vi "Global Schedule Selector.vi"(6 "Scheduler In":refnum<class "Scheduler.lvclass">, 7 "Objective":T1, 8 "error in (no error)":errorcluster, 9 "Reorder?":bool, 10 "Schedule in":u16[](array[numeric]), 11 "OSSP_Problem in":refnum<class "OSSP_Problem.lvclass">) -> (0 "error out":errorcluster, 1 "Total Tardiness or Makespan (U16)":u16, 2 "Schedule out":u16[](array[numeric]), 3 "OSSP_Problem out":refnum<class "OSSP_Problem.lvclass">, 4 "Scheduler out":refnum<class "Scheduler.lvclass">)   [LabVIEW 2013]
uses:
  Classes/OSSP_Problem.lvclass
  GA/Controls/Objective.ctl
  Classes/Scheduler.lvclass
  Classes/Scheduler.lvclass/Scheduler.ctl
  Classes/OSSP_Problem.lvclass/OSSP_Problem.ctl
  Classes/Scheduler_Class/Operation to Machine Job Tuple.vi
  Classes/Scheduler_Class/Prins FIFO Scheduler Methods and Controls/Prins FIFO Scheduler.vi
  Classes/Scheduler_Class/Prins FIFO Scheduler Methods and Controls/Methods/Calculate Final Completion Times of Jobs.vi
  Classes/Scheduler_Class/Prins FIFO Scheduler Methods and Controls/Methods/Reorder Schedule(Prins FIFO) based on Start Times.vi
  Classes/Scheduler_Class/Modified GT Active Scheduler/GT Find Subset of Operations.vi
  Classes/Scheduler_Class/Modified GT Active Scheduler/Select Operation to Schedule Based on Rule.vi
  Classes/Scheduler_Class/Prins FIFO Scheduler Methods and Controls/Methods/UpdateMachineGaps.vi
  Classes/Scheduler_Class/Prins FIFO Scheduler Methods and Controls/Methods/UpdateJobGaps.vi
  Classes/Scheduler_Class/Prins FIFO Scheduler Methods and Controls/Methods/Find Intersecting Gaps.vi
  Classes/Scheduler_Class/GT Algorithm Find M_ok and J_ok.vi
  Classes/Scheduler_Class/Prins FIFO Scheduler Methods and Controls/Methods/Transform to Plain Job and Machine Gaps Array.vi
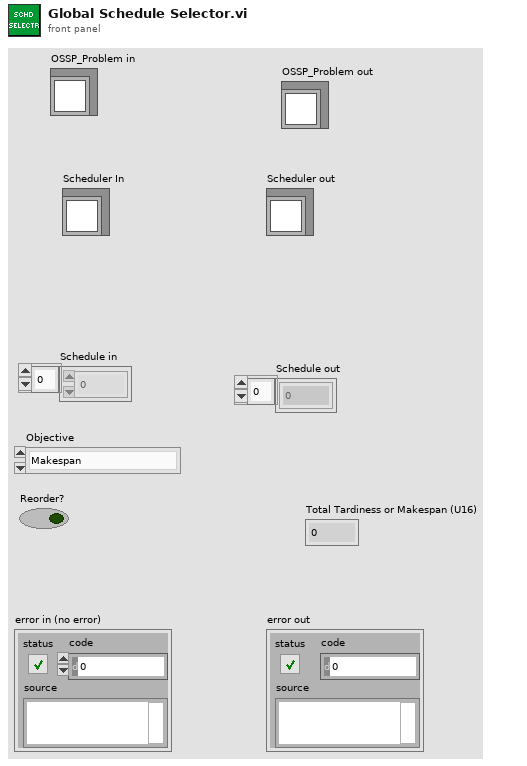
[diagram p1: front panel]
types:
  T1 = typedef "Objective.ctl" = enum16{"Makespan", "Total Tardiness"}
  T2 = typedef "Scheduler Type.ctl" = enum16{"Non Delay Scheduler", "GT Active Scheduler", "My Faulty Scheduler", "Prins FIFO Scheduler", "SemiActive Scheduler", "Modified GT Scheduler"}
  T3 = typedef "Scheduler.lvclass/Operation Selection Rule from Subset to Schedule.ctl" = enum16{"First Operation in Order", "SPT", "EDD", "MDD"}
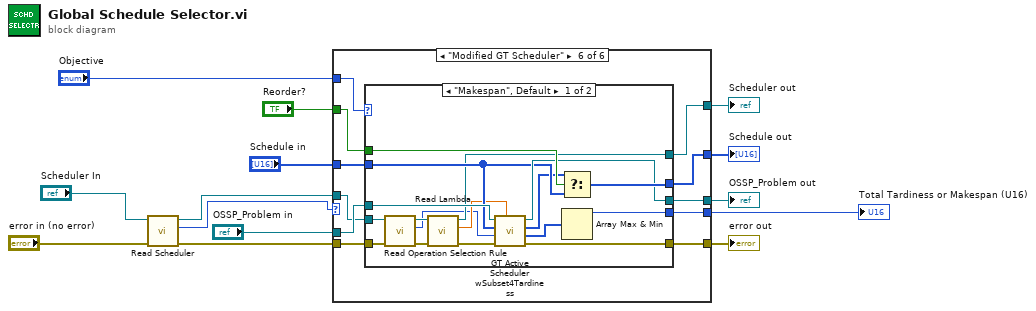
[diagram p0: block diagram]
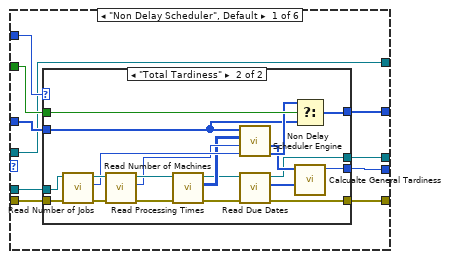
[diagram p2: hidden frame]
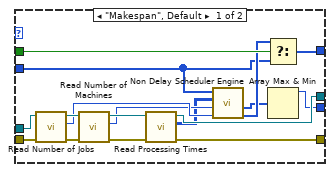
[diagram p3: hidden frame]
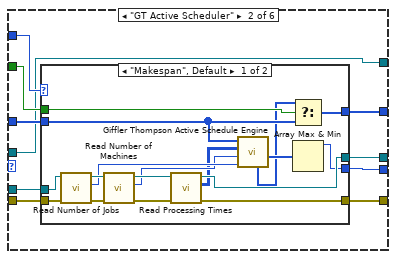
[diagram p4: hidden frame]
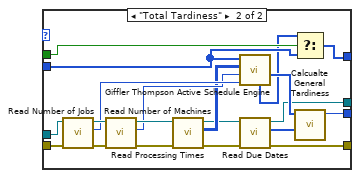
[diagram p5: hidden frame]
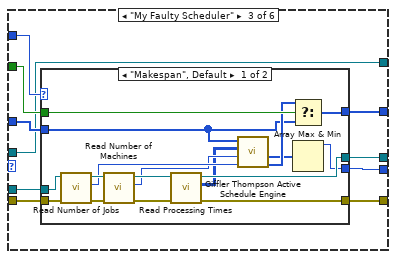
[diagram p6: hidden frame]
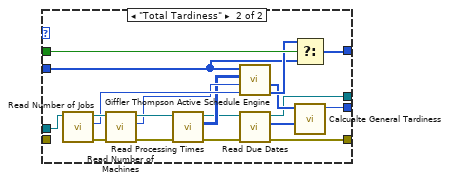
[diagram p7: hidden frame]
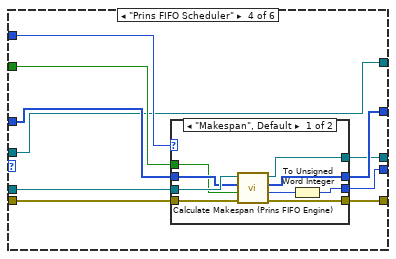
[diagram p8: hidden frame]
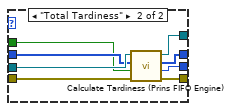
[diagram p9: hidden frame]
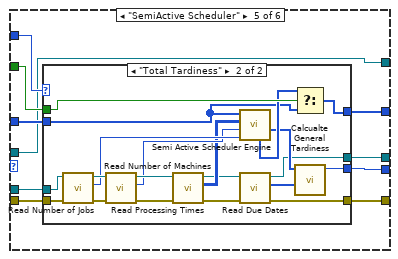
[diagram p10: hidden frame]
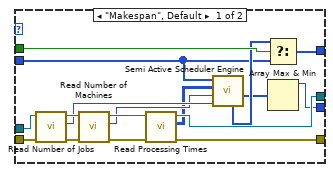
[diagram p11: hidden frame]
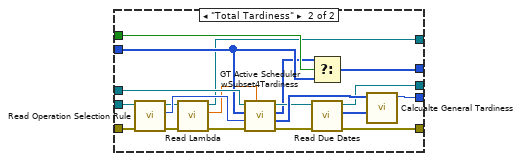
[diagram p12: hidden frame]
diagram:
  n1 = call "Read Scheduler.vi"("error in (no error)"="error in (no error)", "Scheduler in"="Scheduler In") -> ("error out"=w4:errorcluster, "Scheduler"=w1:T2, "Scheduler out"=w2:refnum<class "Scheduler.lvclass">)  [unwired: 7 in]
  n2 = case shown="\"Modified GT Scheduler\"" w1 {
    tunnel: [w16 w66 w111 w164 w184 w232] -> w7
    tunnel: "Schedule in" -> [w19 w69 w117 w163 w190 w238]
    tunnel: [w17 w65 w112 w162 w185 w233] -> w9
    tunnel: "Objective" -> [w24 w63 w115 w161 w189 w237]
    tunnel: "Reorder?" -> [w18 w68 w114 w160 w187 w235]
    tunnel: [w22 w64 w110 w159 w183 w231] -> w12
    tunnel: "OSSP_Problem in" -> [w23 w70 w118 w158 w191 w239]
    tunnel: w4 -> [w21 w71 w116 w157 w188 w236]
    tunnel: [w20 w67 w113 w156 w186 w234] -> w14
    tunnel: w2 -> [w15 w62 w109 w155 w182 w230]
    tunnel: [w15 w62 w109 w155 w182 w229] -> w6
    frame "Non Delay Scheduler", Default {
      n3 = case shown="\"Total Tardiness\"" w24 {
        tunnel: w23 -> [w41 w61]
        tunnel: [w38 w45] -> w22
        tunnel: w21 -> [w37 w58]
        tunnel: [w34 w44] -> w20
        tunnel: w19 -> [w28 w50]
        tunnel: w18 -> [w30 w52]
        tunnel: [w27 w49] -> w17
        tunnel: [w25 w42] -> w16
        frame "Makespan", Default {
          n4 = call "Read Number of Jobs.vi"("error in (no error)"=w37, "OSSP_Problem in"=w41) -> ("error out"=w36:errorcluster, "Number of Jobs"=w33:i32, "OSSP_Problem out"=w40:refnum<class "OSSP_Problem.lvclass">)  [unwired: 7 in]
          n5 = call "Read Number of Machines.vi"("error in (no error)"=w36, "OSSP_Problem in"=w40) -> ("error out"=w35:errorcluster, "Number of Machines"=w32:i32, "OSSP_Problem out"=w39:refnum<class "OSSP_Problem.lvclass">)  [unwired: 7 in]
          n6 = call "Read Processing Times.vi"("error in (no error)"=w35, "OSSP_Problem in"=w39) -> ("error out"=w34:errorcluster, "Processing Times"=w31:u16[][], "OSSP_Problem out"=w38:refnum<class "OSSP_Problem.lvclass">)  [unwired: 7 in]
          n7 = call "Non Delay Scheduler Engine.vi"("Number of  Jobs"=w33, "Number of Machines"=w32, "Processing Times"=w31, "Schedule"=w28) -> ("Reordered Schedule"=w29:u16[], "Job Completion Times"=w26:u16[])  [unwired: 2 in, 4 out]
          n8 = Select(t=w29, s=w30, f=w28) -> (s? t:f=w27:u16[])
          n9 = Array Max & Min(array=w26) -> (max value=w25:u16)  [unwired: 3 out]
        }
        frame "Total Tardiness" {
          n10 = call "Read Number of Jobs.vi"("error in (no error)"=w58, "OSSP_Problem in"=w61) -> ("error out"=w57:errorcluster, "Number of Jobs"=w55:i32, "OSSP_Problem out"=w60:refnum<class "OSSP_Problem.lvclass">)  [unwired: 7 in]
          n11 = call "Read Number of Machines.vi"("error in (no error)"=w57, "OSSP_Problem in"=w60) -> ("error out"=w56:errorcluster, "Number of Machines"=w54:i32, "OSSP_Problem out"=w59:refnum<class "OSSP_Problem.lvclass">)  [unwired: 7 in]
          n12 = call "Read Processing Times.vi"("error in (no error)"=w56, "OSSP_Problem in"=w59) -> ("error out"=w47:errorcluster, "Processing Times"=w53:u16[][], "OSSP_Problem out"=w46:refnum<class "OSSP_Problem.lvclass">)  [unwired: 7 in]
          n13 = call "Non Delay Scheduler Engine.vi"("Number of  Jobs"=w55, "Number of Machines"=w54, "Processing Times"=w53, "Schedule"=w50) -> ("Reordered Schedule"=w51:u16[], "Job Completion Times"=w48:u16[])  [unwired: 2 in, 4 out]
          n14 = call "Read Due Dates.vi"("error in (no error)"=w47, "OSSP_Problem in"=w46) -> ("error out"=w44:errorcluster, "Due Dates"=w43:u16[], "OSSP_Problem out"=w45:refnum<class "OSSP_Problem.lvclass">)  [unwired: 7 in]
          n15 = Select(t=w51, s=w52, f=w50) -> (s? t:f=w49:u16[])
          n16 = call "Calcualte General Tardiness.vi"("Due Dates"=w43, "Job Completion Times"=w48) -> ("Total Tardiness (U16)"=w42:u16)  [unwired: 9 in]
        }
      }
    }
    frame "GT Active Scheduler" {
      n17 = case shown="\"Makespan\", Default" w63 {
        tunnel: w70 -> [w88 w108]
        tunnel: [w85 w93] -> w64
        tunnel: w71 -> [w84 w105]
        tunnel: [w81 w92] -> w67
        tunnel: w69 -> [w76 w98]
        tunnel: w68 -> [w77 w99]
        tunnel: [w75 w97] -> w65
        tunnel: [w73 w90] -> w66
        frame "Makespan", Default {
          n18 = call "Read Number of Jobs.vi"("error in (no error)"=w84, "OSSP_Problem in"=w88) -> ("error out"=w83:errorcluster, "Number of Jobs"=w80:i32, "OSSP_Problem out"=w87:refnum<class "OSSP_Problem.lvclass">)  [unwired: 7 in]
          n19 = call "Read Number of Machines.vi"("error in (no error)"=w83, "OSSP_Problem in"=w87) -> ("error out"=w82:errorcluster, "Number of Machines"=w79:i32, "OSSP_Problem out"=w86:refnum<class "OSSP_Problem.lvclass">)  [unwired: 7 in]
          n20 = call "Read Processing Times.vi"("error in (no error)"=w82, "OSSP_Problem in"=w86) -> ("error out"=w81:errorcluster, "Processing Times"=w78:u16[][], "OSSP_Problem out"=w85:refnum<class "OSSP_Problem.lvclass">)  [unwired: 7 in]
          n21 = call "Giffler Thompson Active Schedule Engine.vi"("Number of  Jobs"=w80, "Number of Machines"=w79, "Processing Times"=w78, "Schedule In"=w76) -> ("Job Completion Times"=w74:u16[], "Ordered Schedule Out"=w72:u16[])  [unwired: 3 in, 3 out]
          n22 = Select(t=w72, s=w77, f=w76) -> (s? t:f=w75:u16[])
          n23 = Array Max & Min(array=w74) -> (max value=w73:u16)  [unwired: 3 out]
        }
        frame "Total Tardiness" {
          n24 = call "Read Number of Jobs.vi"("error in (no error)"=w105, "OSSP_Problem in"=w108) -> ("error out"=w104:errorcluster, "Number of Jobs"=w102:i32, "OSSP_Problem out"=w107:refnum<class "OSSP_Problem.lvclass">)  [unwired: 7 in]
          n25 = call "Read Number of Machines.vi"("error in (no error)"=w104, "OSSP_Problem in"=w107) -> ("error out"=w103:errorcluster, "Number of Machines"=w101:i32, "OSSP_Problem out"=w106:refnum<class "OSSP_Problem.lvclass">)  [unwired: 7 in]
          n26 = call "Read Processing Times.vi"("error in (no error)"=w103, "OSSP_Problem in"=w106) -> ("error out"=w95:errorcluster, "Processing Times"=w100:u16[][], "OSSP_Problem out"=w94:refnum<class "OSSP_Problem.lvclass">)  [unwired: 7 in]
          n27 = call "Giffler Thompson Active Schedule Engine.vi"("Number of  Jobs"=w102, "Number of Machines"=w101, "Processing Times"=w100, "Schedule In"=w98) -> ("Job Completion Times"=w96:u16[], "Ordered Schedule Out"=w89:u16[])  [unwired: 3 in, 3 out]
          n28 = call "Read Due Dates.vi"("error in (no error)"=w95, "OSSP_Problem in"=w94) -> ("error out"=w92:errorcluster, "Due Dates"=w91:u16[], "OSSP_Problem out"=w93:refnum<class "OSSP_Problem.lvclass">)  [unwired: 7 in]
          n29 = Select(t=w89, s=w99, f=w98) -> (s? t:f=w97:u16[])
          n30 = call "Calcualte General Tardiness.vi"("Due Dates"=w91, "Job Completion Times"=w96) -> ("Total Tardiness (U16)"=w90:u16)  [unwired: 9 in]
        }
      }
    }
    frame "My Faulty Scheduler" {
      n31 = case shown="\"Makespan\", Default" w115 {
        tunnel: w118 -> [w135 w154]
        tunnel: [w132 w139] -> w110
        tunnel: [w129 w138] -> w113
        tunnel: w117 -> [w123 w144]
        tunnel: w114 -> [w125 w146]
        tunnel: [w122 w143] -> w112
        tunnel: [w120 w136] -> w111
        tunnel: w116 -> [w119 _]
        frame "Makespan", Default {
          n32 = call "Read Number of Jobs.vi"("error in (no error)"=w119, "OSSP_Problem in"=w135) -> ("error out"=w131:errorcluster, "Number of Jobs"=w128:i32, "OSSP_Problem out"=w134:refnum<class "OSSP_Problem.lvclass">)  [unwired: 7 in]
          n33 = call "Read Number of Machines.vi"("error in (no error)"=w131, "OSSP_Problem in"=w134) -> ("error out"=w130:errorcluster, "Number of Machines"=w127:i32, "OSSP_Problem out"=w133:refnum<class "OSSP_Problem.lvclass">)  [unwired: 7 in]
          n34 = call "Read Processing Times.vi"("error in (no error)"=w130, "OSSP_Problem in"=w133) -> ("error out"=w129:errorcluster, "Processing Times"=w126:u16[][], "OSSP_Problem out"=w132:refnum<class "OSSP_Problem.lvclass">)  [unwired: 7 in]
          n35 = call "Giffler Thompson Active Schedule Engine.vi"("Number of  Jobs"=w128, "Number of Machines"=w127, "Processing Times"=w126, "Schedule In"=w123) -> ("Machine Completion Times"=w124:u16[], "Job Completion Times"=w121:u16[])  [unwired: 3 in, 3 out]
          n36 = Select(t=w124, s=w125, f=w123) -> (s? t:f=w122:u16[])
          n37 = Array Max & Min(array=w121) -> (max value=w120:u16)  [unwired: 3 out]
        }
        frame "Total Tardiness" {
          n38 = call "Read Number of Jobs.vi"("OSSP_Problem in"=w154) -> ("error out"=w151:errorcluster, "Number of Jobs"=w149:i32, "OSSP_Problem out"=w153:refnum<class "OSSP_Problem.lvclass">)  [unwired: 8 in]
          n39 = call "Read Number of Machines.vi"("error in (no error)"=w151, "OSSP_Problem in"=w153) -> ("error out"=w150:errorcluster, "Number of Machines"=w148:i32, "OSSP_Problem out"=w152:refnum<class "OSSP_Problem.lvclass">)  [unwired: 7 in]
          n40 = call "Read Processing Times.vi"("error in (no error)"=w150, "OSSP_Problem in"=w152) -> ("error out"=w141:errorcluster, "Processing Times"=w147:u16[][], "OSSP_Problem out"=w140:refnum<class "OSSP_Problem.lvclass">)  [unwired: 7 in]
          n41 = call "Giffler Thompson Active Schedule Engine.vi"("Number of  Jobs"=w149, "Number of Machines"=w148, "Processing Times"=w147, "Schedule In"=w144) -> ("Machine Completion Times"=w145:u16[], "Job Completion Times"=w142:u16[])  [unwired: 3 in, 3 out]
          n42 = call "Read Due Dates.vi"("error in (no error)"=w141, "OSSP_Problem in"=w140) -> ("error out"=w138:errorcluster, "Due Dates"=w137:u16[], "OSSP_Problem out"=w139:refnum<class "OSSP_Problem.lvclass">)  [unwired: 7 in]
          n43 = Select(t=w145, s=w146, f=w144) -> (s? t:f=w143:u16[])
          n44 = call "Calcualte General Tardiness.vi"("Due Dates"=w137, "Job Completion Times"=w142) -> ("Total Tardiness (U16)"=w136:u16)  [unwired: 9 in]
        }
      }
    }
    frame "Prins FIFO Scheduler" {
      n45 = case shown="\"Makespan\", Default" w161 {
        tunnel: [w172 w180] -> w164
        tunnel: w163 -> [w168 w177]
        tunnel: [w173 w181] -> w162
        tunnel: w160 -> [w167 w176]
        tunnel: w158 -> [w169 w179]
        tunnel: [w166 w178] -> w159
        tunnel: w157 -> [w170 w175]
        tunnel: [w165 w174] -> w156
        frame "Makespan", Default {
          n46 = call "Calculate Makespan (Prins FIFO Engine).vi"("error in (no error)"=w170, "Reorder?"=w167, "Schedule In"=w168, "OSSP_Problem in"=w169) -> ("error out"=w165:errorcluster, "Makespan"=w171:i32, "Schedule Out"=w173:u16[], "OSSP_Problem out"=w166:refnum<class "OSSP_Problem.lvclass">)  [unwired: 4 in]
          n47 = To Unsigned Word Integer(number=w171) -> (unsigned 16bit integer=w172:u16)
        }
        frame "Total Tardiness" {
          n48 = call "Calculate Tardiness (Prins FIFO Engine).vi"("error in (no error)"=w175, "Reorder?"=w176, "Schedule In"=w177, "OSSP_Problem in"=w179) -> ("error out"=w174:errorcluster, "Tardiness(Prins FIFO Engine)"=w180:u16, "Schedule Out"=w181:u16[], "OSSP_Problem out"=w178:refnum<class "OSSP_Problem.lvclass">)  [unwired: 3 in, 1 out]
        }
      }
    }
    frame "SemiActive Scheduler" {
      n49 = case shown="\"Total Tardiness\"" w189 {
        tunnel: w191 -> [w208 w228]
        tunnel: [w205 w212] -> w183
        tunnel: w188 -> [w204 w225]
        tunnel: [w201 w211] -> w186
        tunnel: w190 -> [w195 w217]
        tunnel: w187 -> [w197 w219]
        tunnel: [w194 w216] -> w185
        tunnel: [w192 w209] -> w184
        frame "Makespan", Default {
          n50 = call "Read Number of Jobs.vi"("error in (no error)"=w204, "OSSP_Problem in"=w208) -> ("error out"=w203:errorcluster, "Number of Jobs"=w200:i32, "OSSP_Problem out"=w207:refnum<class "OSSP_Problem.lvclass">)  [unwired: 7 in]
          n51 = call "Read Number of Machines.vi"("error in (no error)"=w203, "OSSP_Problem in"=w207) -> ("error out"=w202:errorcluster, "Number of Machines"=w199:i32, "OSSP_Problem out"=w206:refnum<class "OSSP_Problem.lvclass">)  [unwired: 7 in]
          n52 = call "Read Processing Times.vi"("error in (no error)"=w202, "OSSP_Problem in"=w206) -> ("error out"=w201:errorcluster, "Processing Times"=w198:u16[][], "OSSP_Problem out"=w205:refnum<class "OSSP_Problem.lvclass">)  [unwired: 7 in]
          n53 = call "Semi Active Scheduler Engine.vi"("Number of  Jobs"=w200, "Number of Machines"=w199, "Processing Times"=w198, "Schedule"=w195) -> ("Job Completion Times"=w193:u16[], "Machine Completion Times"=w196:u16[])  [unwired: 3 in, 3 out]
          n54 = Select(t=w196, s=w197, f=w195) -> (s? t:f=w194:u16[])
          n55 = Array Max & Min(array=w193) -> (max value=w192:u16)  [unwired: 3 out]
        }
        frame "Total Tardiness" {
          n56 = call "Read Number of Jobs.vi"("error in (no error)"=w225, "OSSP_Problem in"=w228) -> ("error out"=w224:errorcluster, "Number of Jobs"=w222:i32, "OSSP_Problem out"=w227:refnum<class "OSSP_Problem.lvclass">)  [unwired: 7 in]
          n57 = call "Read Number of Machines.vi"("error in (no error)"=w224, "OSSP_Problem in"=w227) -> ("error out"=w223:errorcluster, "Number of Machines"=w221:i32, "OSSP_Problem out"=w226:refnum<class "OSSP_Problem.lvclass">)  [unwired: 7 in]
          n58 = call "Read Processing Times.vi"("error in (no error)"=w223, "OSSP_Problem in"=w226) -> ("error out"=w214:errorcluster, "Processing Times"=w220:u16[][], "OSSP_Problem out"=w213:refnum<class "OSSP_Problem.lvclass">)  [unwired: 7 in]
          n59 = call "Semi Active Scheduler Engine.vi"("Number of  Jobs"=w222, "Number of Machines"=w221, "Processing Times"=w220, "Schedule"=w217) -> ("Job Completion Times"=w215:u16[], "Machine Completion Times"=w218:u16[])  [unwired: 3 in, 3 out]
          n60 = call "Read Due Dates.vi"("error in (no error)"=w214, "OSSP_Problem in"=w213) -> ("error out"=w211:errorcluster, "Due Dates"=w210:u16[], "OSSP_Problem out"=w212:refnum<class "OSSP_Problem.lvclass">)  [unwired: 7 in]
          n61 = Select(t=w218, s=w219, f=w217) -> (s? t:f=w216:u16[])
          n62 = call "Calcualte General Tardiness.vi"("Due Dates"=w210, "Job Completion Times"=w215) -> ("Total Tardiness (U16)"=w209:u16)  [unwired: 9 in]
        }
      }
    }
    frame "Modified GT Scheduler" {
      n63 = case shown="\"Makespan\", Default" w237 {
        tunnel: w239 -> [w253 w273]
        tunnel: [w252 w269] -> w231
        tunnel: w236 -> [w242 w263]
        tunnel: [w251 w267] -> w234
        tunnel: w238 -> [w250 w272]
        tunnel: w235 -> [w256 w276]
        tunnel: [w255 w275] -> w233
        tunnel: [w254 w274] -> w232
        tunnel: w230 -> [w244 w264]
        tunnel: [w245 w259] -> w229
        frame "Makespan", Default {
          n64 = call "Read Operation Selection Rule.vi"("error in (no error)"=w242, "Scheduler in"=w244) -> ("error out"=w241:errorcluster, "Operation Seletion Rule"=w240:T3, "Scheduler out"=w243:refnum<class "Scheduler.lvclass">)  [unwired: 7 in]
          n65 = call "Read Lambda.vi"("error in (no error)"=w241, "Scheduler in"=w243) -> ("error out"=w247:errorcluster, "Lambda"=w246:dbl, "Scheduler out"=w245:refnum<class "Scheduler.lvclass">)  [unwired: 7 in]
          n66 = call "GT Active Scheduler wSubset4Tardiness.vi"("Lambda"=w246, "error in (no error)"=w247, "Operation Selection Rule"=w240, "Schedule In"=w250, "OSSP_Problem.lvclass"=w253) -> ("error out"=w251:errorcluster, "Job Completion Times"=w249:u16[], "Ordered Schedule Out"=w248:u16[], "OSSP_Problem out"=w252:refnum<class "OSSP_Problem.lvclass">)  [unwired: 1 in, 2 out]
          n67 = Select(t=w248, s=w256, f=w250) -> (s? t:f=w255:u16[])
          n68 = Array Max & Min(array=w249) -> (max value=w254:u16)  [unwired: 3 out]
        }
        frame "Total Tardiness" {
          n69 = call "Read Operation Selection Rule.vi"("error in (no error)"=w263, "Scheduler in"=w264) -> ("error out"=w261:errorcluster, "Operation Seletion Rule"=w262:T3, "Scheduler out"=w260:refnum<class "Scheduler.lvclass">)  [unwired: 7 in]
          n70 = call "Read Lambda.vi"("error in (no error)"=w261, "Scheduler in"=w260) -> ("error out"=w257:errorcluster, "Lambda"=w258:dbl, "Scheduler out"=w259:refnum<class "Scheduler.lvclass">)  [unwired: 7 in]
          n71 = call "GT Active Scheduler wSubset4Tardiness.vi"("Lambda"=w258, "error in (no error)"=w257, "Operation Selection Rule"=w262, "Schedule In"=w272, "OSSP_Problem.lvclass"=w273) -> ("error out"=w268:errorcluster, "Job Completion Times"=w271:u16[], "Ordered Schedule Out"=w266:u16[], "OSSP_Problem out"=w270:refnum<class "OSSP_Problem.lvclass">)  [unwired: 1 in, 2 out]
          n72 = Select(t=w266, s=w276, f=w272) -> (s? t:f=w275:u16[])
          n73 = call "Read Due Dates.vi"("error in (no error)"=w268, "OSSP_Problem in"=w270) -> ("error out"=w267:errorcluster, "Due Dates"=w265:u16[], "OSSP_Problem out"=w269:refnum<class "OSSP_Problem.lvclass">)  [unwired: 7 in]
          n74 = call "Calcualte General Tardiness.vi"("Due Dates"=w265, "Job Completion Times"=w271) -> ("Total Tardiness (U16)"=w274:u16)  [unwired: 9 in]
        }
      }
    }
  }
  "error out" <- w14
  "OSSP_Problem out" <- w12
  "Schedule out" <- w9
  "Total Tardiness or Makespan (U16)" <- w7
  "Scheduler out" <- w6
